vi "PXDAC4800_SetDacSampleSizeXD48.vi"(2 "Value":u32, 3 "Handle":u32) -> (0 "Status":i32, 1 "Handle out":u32)   [LabVIEW 2016]
uses:
  PXDAC4800.dll
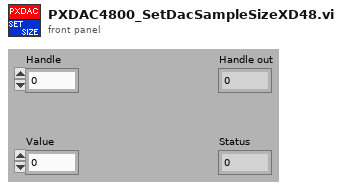
[diagram p1: front panel]
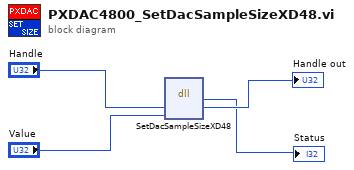
[diagram p0: block diagram]
diagram:
  n1 = dll-call lib="PXDAC4800.dll" fn="SetDacSampleSizeXD48"("Handle"="Handle", "val"="Value") -> (→"Status":i32, "Handle"=→"Handle out":u32)  [unwired: 4 in, 2 out]
